vi "send.vi"(0 "HGF_Occurrence":refnum<class "HGF_Occurrence.lvclass">, 2 "Object":refnum<class>, 3 "timeout in ms (-1)":i32, 5 "error in (no error)":errorcluster, 9 "mode (Queue)":bool) -> (14 "dup HGF_Occurrence":refnum<class "HGF_Occurrence.lvclass">, 17 "timed out?":bool, 19 "error out":errorcluster)   [LabVIEW 2014, in "HGF_BaseClasses.lvlib" / "HGF_Occurrence.lvclass"]
doc: "Send an object.\n\nHint: This is a dynamic dispatch VI to be implemented by the child class."
uses:
  HGF_Occurrence.lvclass
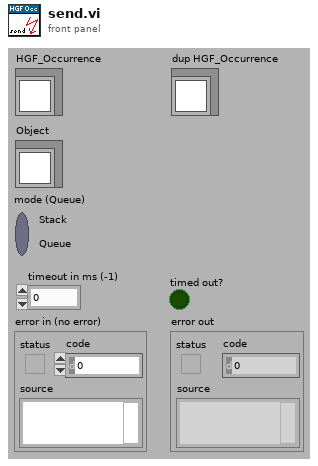
[diagram p1: front panel]
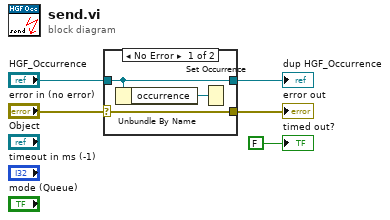
[diagram p0: block diagram]
diagram:
  n1 = case shown="No Error" "error in (no error)" {
    selector: "error in (no error)" -> [w8 w10]
    tunnel: [w7 w9] -> w5
    tunnel: "HGF_Occurrence" -> [w7 w9]
    tunnel: [w8 w10] -> w1
    frame No Error {
      n2 = Unbundle By Name(w7) -> ("occurrence"=w6:refnum<k4>)
      n3 = Set Occurrence(w6) -> ()
    }
    frame Error {
    }
  }
  "error out" <- w1
  "dup HGF_Occurrence" <- w5
  "timed out?" <- FALSE ("timed out?")
